vi "Camera.vi"(0 "Camera in":refnum<class "Camera.lvclass">, 1 "Stop":bool, 4 "BCG Image Processing":T3={"Brightness"=128.0, "Contrast"=45.0, "Gamma"=1.0} {"Brightness" scale=0.0..400.0; "Contrast" scale=0.0..90.0; "Gamma" scale=0.005..5.0}, 5 "error in (no error)":errorcluster, 6 "Machine Vision":T5, 7 "Camera settings":T2={"Gamma"=1.0, "Gain"=7, "Sharpness"=0, "Contrast"=0.009999999999999995, "Exposure"=0.0004073180282999787} {"Exposure" min=0.000244140625 max=0.5 scale=0.0002..0.5; "Contrast" min=0.0 max=1.0 scale=0.001..1.0; "Sharpness" min=0 max=2 step=1 scale=0.0..2.0; "Gain" min=0 max=100 step=1 scale=0.1..100.0; "Gamma" min=0.01 max=10.0 scale=0.01..10.0}, 10 "Material":T4, 12 "Loop 0":bool, 13 "Override presets":bool) -> (11 "Radius (Real-World)":dbl, 14 "Camera out":refnum<class "Camera.lvclass">, 15 "Average Strength":dbl, 16 "Global Report":T1 {"Mean Value" format="%.2f"; "%" format="%.2f"; "Area (calibrated)" format="%.2f"; "Maximal Value" format="%.2f"; "Minimal Value" format="%.2f"; "Standard Variation" format="%.2f"}, 17 "Image":T6(plugin-control), 18 "Camera":dbl[](array[numeric]), 19 "error out":errorcluster)   [LabVIEW 2021, in "Camera.lvclass"]
uses:
  Camera.lvclass
  Machine Vision.ctl
  Material.ctl
  Image processing.ctl
  Camera settings.ctl
  <vilib>/Utility/file.llb/Read Delimited Spreadsheet (string).vi
  <vilib>/vision/NI_Vision_Development_Module.lvlib
panel:
  out "Y":sgl
  out "X":sgl
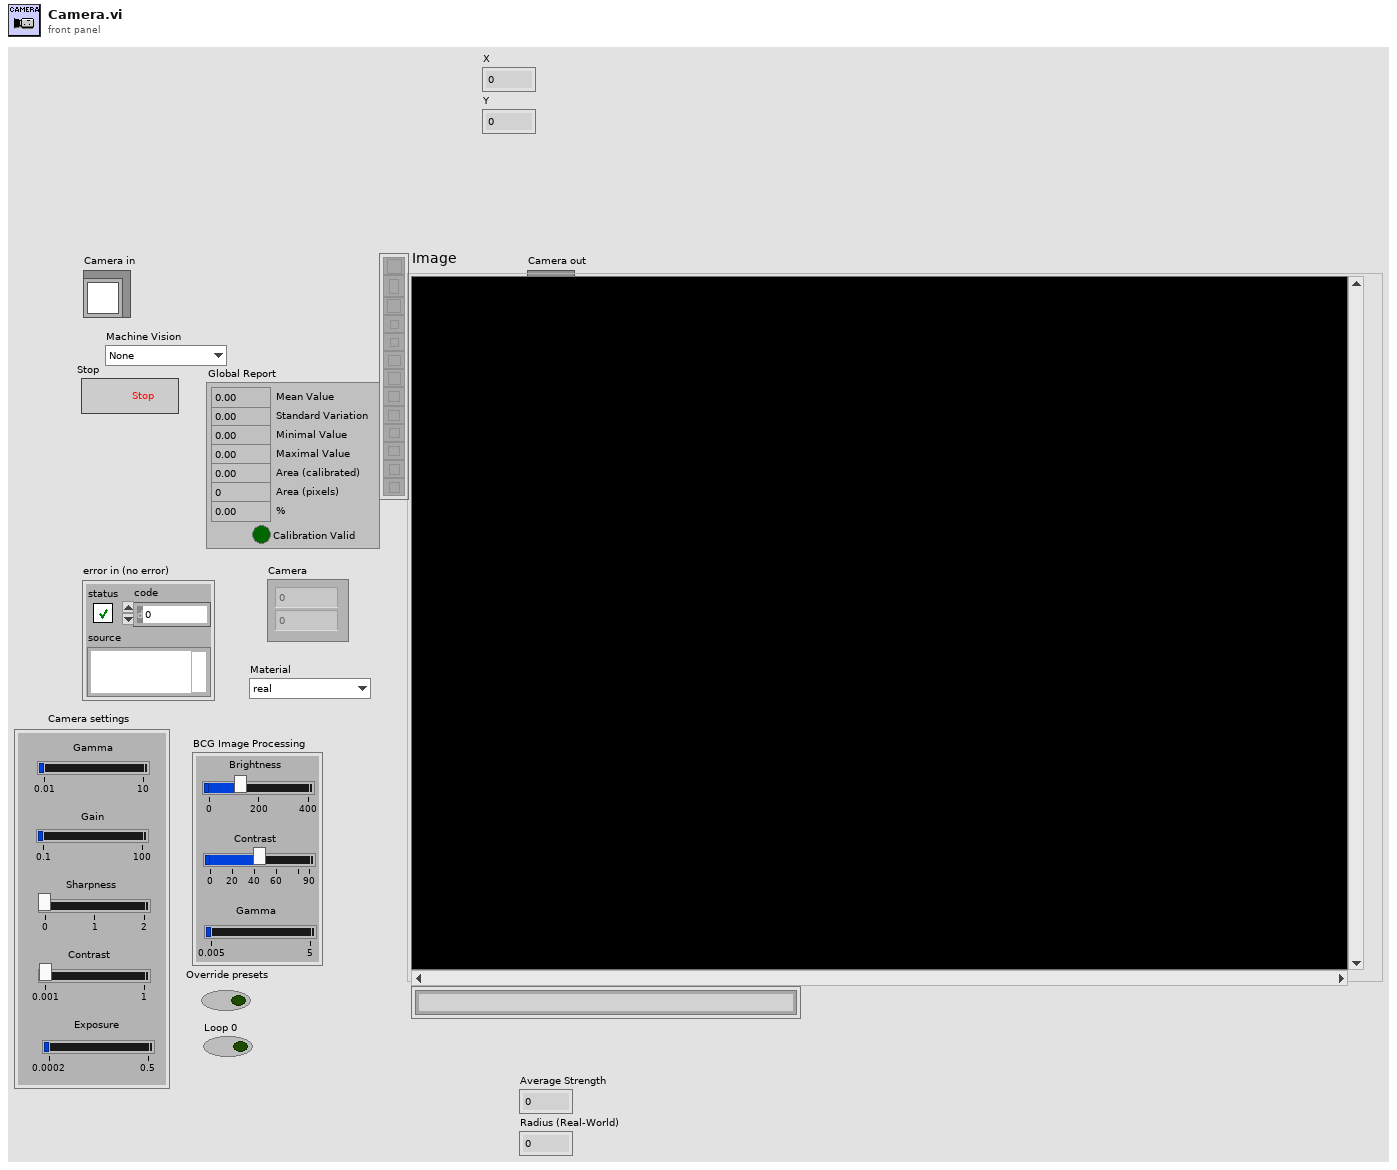
[diagram p1: front panel]
types:
  T1 = cluster{"Mean Value":sgl, "Standard Variation":sgl, "Minimal Value":sgl, "Maximal Value":sgl, "Area (calibrated)":sgl, "Area (pixels)":u32, "%":sgl, "Calibration Valid":bool}
  T2 = typedef "Camera.lvclass/Camera settings.ctl" = cluster{"Gamma":dbl, "Gain":i64, "Sharpness":i64, "Contrast":dbl, "Exposure":dbl}
  T3 = typedef "Camera.lvclass/Image processing.ctl" = cluster{"Brightness":sgl, "Contrast":sgl, "Gamma":sgl}
  T4 = typedef "Camera.lvclass/Material.ctl" = enum16{"real", "dummy", "PETG"}
  T5 = typedef "Camera.lvclass/Machine Vision.ctl" = enum16{"None", "Tray Fiducials", "Sensor Fiducials", "HPK Silicon", "Partial Hexaboard", "Partial Hexaboard Test", "100um dot", "Hexaboard", "Corner (TL, BR)", "Corner (BL, TR)", "V3 Sensor Cross", "V3 Sensor Circle", "test"}
  T6 = typedef "IMAQ Image.ctl" = refnum<image>
  T7 = typedef "File Paths.ctl" = cluster{"Glue Pattern Folder":path, "Carrier Tray Folder":path, "Pick Up Tool Fixture Folder":path, "Components Folder":path, "Bellows Tool Offset.txt":path, "Pick Up Tool Offset.txt":path, "Dispense Tip Offset.txt":path, "Log Files":path, "Gantry Assembly Map.txt":path, "Syringe and offset map.txt":path, "Controllers Folder":path, "Local dbase config":path}
  T8 = cluster{"Center (Pixels)":cluster{"X":sgl, "Y":sgl}, "Radius (Pixels)":dbl, "Center (Real-World)":cluster{"X":sgl, "Y":sgl}, "Radius (Real-World)":dbl, "Roundness (Real-World)":dbl, "Average Strength":dbl, "Average SNR (dB)":dbl}
  T9 = typedef "Edge New.ctl" = cluster{"Location (Pixel)":cluster{"X":sgl, "Y":sgl}, "Location (Real-World)":cluster{"X":sgl, "Y":sgl}, "Distance (Pixel)":dbl, "Distance (Real-World)":dbl, "Strength":dbl, "Noise":dbl, "Rising?":bool}
  T10 = cluster{"output string":sgl, "output string":sgl}
  T11 = typedef "ROI Descriptor" = cluster{"Global Rectangle":i32[], "Contours":cluster{"ID":enum32{"External", "Internal"}, "Type":u32, "Coordinates":i32[]}[]}
  T12 = typedef "Image Type" = u32
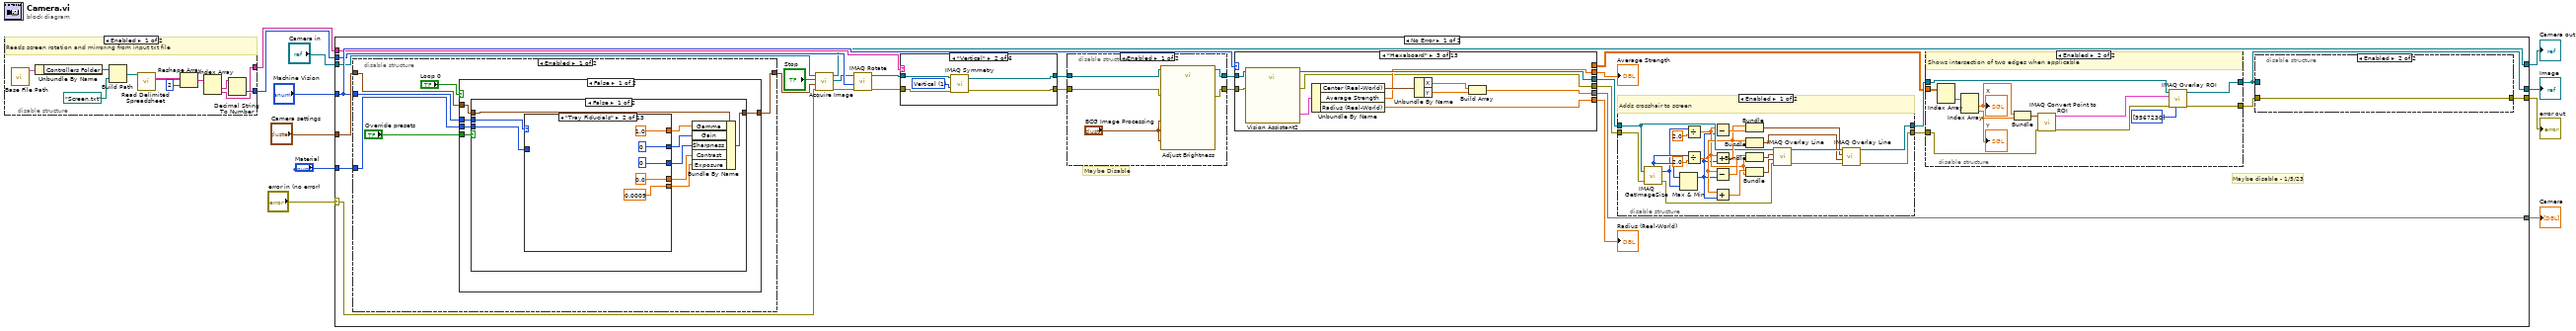
[diagram p0: block diagram]
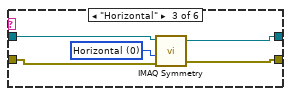
[diagram p4: hidden frame]
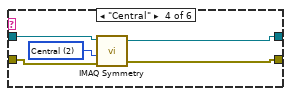
[diagram p5: hidden frame]
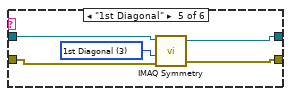
[diagram p6: hidden frame]
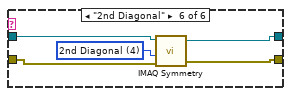
[diagram p7: hidden frame]
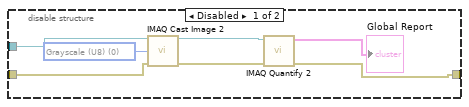
[diagram p8: hidden frame]
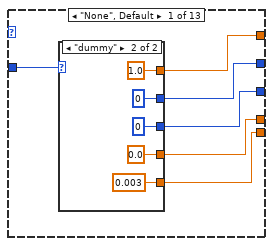
[diagram p12: hidden frame]
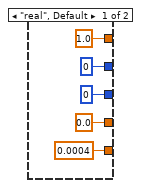
[diagram p13: hidden frame]
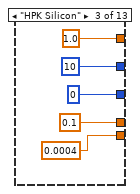
[diagram p14: hidden frame]
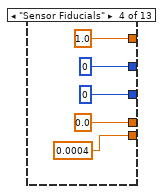
[diagram p15: hidden frame]
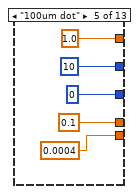
[diagram p16: hidden frame]
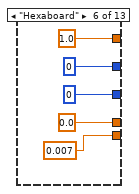
[diagram p17: hidden frame]
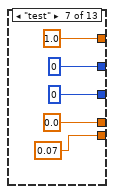
[diagram p18: hidden frame]
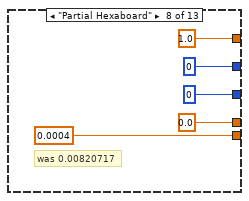
[diagram p19: hidden frame]
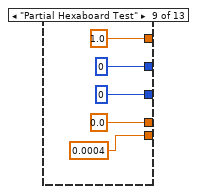
[diagram p20: hidden frame]
diagram:
  n1 = disable-structure shown="Enabled" {
    disable-tunnel: [w13 _] -> w2
    disable-tunnel: [w12 _] -> w1
    frame Enabled {
      # "Reads screen rotation and mirroring from input txt file"
      n2 = call "Base File Path.vi"() -> ("Paths Out"=w21:T7)  [unwired: 11 in]
      n3 = Unbundle By Name(w21) -> ("Controllers Folder"=w20:path)
      n4 = Build Path(base path=w20, name or relative path=path "Screen.txt") -> (appended path=w18:path)
      n5 = call-poly <vilib>:"Read Delimited Spreadsheet.vi"("file path (dialog if empty)"=w18) -> ("all rows"=w17:string[][])  [unwired: 9 in, 5 out]
      n6 = Reshape Array(w17, 2 ("dimension size")) -> (w15:string[])
      n7 = Index Array(array=w15) -> (element #1=w14:string, element #2=w12:string)  [unwired: 2 in]
      n8 = Decimal String To Number(string=w14) -> (number=w13:i32)  [unwired: 2 in, 1 out]
    }
    frame Disabled {
    }
  }
  n9 = case shown="No Error" "error in (no error)" {
    selector: "error in (no error)" -> [w24 w374]
    tunnel: [w31 w374] -> w10
    tunnel: [w27 w373] -> w9
    tunnel: "Camera in" -> [w28 w373]
    tunnel: [w50 _] -> w7
    tunnel: [w33 _] -> w6
    tunnel: "Machine Vision" -> [w48 _]
    tunnel: "Camera settings" -> [w49 _]
    tunnel: "Material" -> [w47 _]
    tunnel: w2 -> [w30 _]
    tunnel: w1 -> [w29 _]
    frame No Error {
      # "Maybe Disable"
      # "Maybe disable - 1/5/23"
      n10 = disable-structure shown="Enabled" {
        disable-tunnel: w48 -> [w136 _]
        disable-tunnel: w49 -> [w135 w235]
        disable-tunnel: [w134 w235] -> w25
        disable-tunnel: w47 -> [w131 _]
        frame Enabled {
          n11 = case shown="False" "Loop 0" {
            tunnel: "Override presets" -> [w141 _]
            tunnel: w136 -> [w140 _]
            tunnel: w135 -> [w139 w234]
            tunnel: [w138 w233] -> w134
            tunnel: w131 -> [w137 _]
            frame False {
              n12 = case shown="False" w141 {
                tunnel: w140 -> [w150 _]
                tunnel: w139 -> [w149 w227]
                tunnel: [w143 w227] -> w138
                tunnel: w137 -> [w142 _]
                frame False {
                  n13 = case shown="\"Tray Fiducials\"" w150 {
                    tunnel: [w155 1.0 ("Gamma::Value") 1.0 ("Gamma::Value") 1.0 ("Gamma::Value") 1.0 ("Gamma::Value") 1.0 ("Gamma::Value") 1.0 ("Gamma::Value") 1.0 ("Gamma::Value") 1.0 ("Gamma::Value") 1.0 ("Gamma::Value") 1.0 ("Gamma::Value") 1.0 ("Gamma::Value") 1.0 ("Gamma::Value")] -> w148
                    tunnel: [w151 i64 0 ("Gain::Value") i64 10 ("Gain::Value") i64 0 ("Gain::Value") i64 10 ("Gain::Value") i64 0 ("Gain::Value") i64 0 ("Gain::Value") i64 0 ("Gain::Value") i64 0 ("Gain::Value") i64 10 ("Gain::Value") i64 0 ("Gain::Value") i64 0 ("Gain::Value") i64 0 ("Gain::Value")] -> w147
                    tunnel: [w152 i64 0 ("Sharpness::Value") i64 0 ("Sharpness::Value") i64 0 ("Sharpness::Value") i64 0 ("Sharpness::Value") i64 0 ("Sharpness::Value") i64 0 ("Sharpness::Value") i64 0 ("Sharpness::Value") i64 0 ("Sharpness::Value") i64 0 ("Sharpness::Value") i64 0 ("Sharpness::Value") i64 0 ("Sharpness::Value") i64 0 ("Sharpness::Value")] -> w146
                    tunnel: [w153 0.0 ("Contrast::Value") 0.1 ("Contrast::Value") 0.0 ("Contrast::Value") 0.1 ("Contrast::Value") 0.0 ("Contrast::Value") 0.0 ("Contrast::Value") 0.0 ("Contrast::Value") 0.0 ("Contrast::Value") 0.075 ("Contrast::Value") 0.0 ("Contrast::Value") 0.0 ("Contrast::Value") 0.0 ("Contrast::Value")] -> w145
                    tunnel: [w154 0.0009 ("Exposure::Value") 0.0004 ("Exposure::Value") 0.0004 ("Exposure::Value") 0.0004 ("Exposure::Value") 0.007 ("Exposure::Value") 0.07 ("Exposure::Value") 0.0004 ("Exposure::Value") 0.0004 ("Exposure::Value") 0.0004 ("Exposure::Value") 0.007 ("Exposure::Value") 0.007 ("Exposure::Value") 0.001 ("Exposure::Value")] -> w144
                    tunnel: w142 -> [w156 _ _ _ _ _ _ _ _ _ _ _ _]
                    frame "None", Default {
                      n14 = case shown="\"dummy\"" w156 {
                        tunnel: [1.0 ("Gamma::Value") 1.0 ("Gamma::Value")] -> w155
                        tunnel: [0.0004 ("Exposure::Value") 0.003 ("Exposure::Value")] -> w154
                        tunnel: [0.0 ("Contrast::Value") 0.0 ("Contrast::Value")] -> w153
                        tunnel: [i64 0 ("Sharpness::Value") i64 0 ("Sharpness::Value")] -> w152
                        tunnel: [i64 0 ("Gain::Value") i64 0 ("Gain::Value")] -> w151
                        frame "real", Default {
                        }
                        frame "dummy" {
                        }
                      }
                    }
                    frame "Tray Fiducials" {
                    }
                    frame "HPK Silicon" {
                    }
                    frame "Sensor Fiducials" {
                    }
                    frame "100um dot" {
                    }
                    frame "Hexaboard" {
                    }
                    frame "test" {
                    }
                    frame "Partial Hexaboard" {
                      # "was 0.00820717"
                    }
                    frame "Partial Hexaboard Test" {
                    }
                    frame "Corner (TL, BR)" {
                    }
                    frame "Corner (BL, TR)" {
                    }
                    frame "V3 Sensor Cross" {
                    }
                    frame "V3 Sensor Circle" {
                    }
                  }
                  n15 = Bundle By Name(cluster=w149, "Gamma"=w148, "Gain"=w147, "Sharpness"=w146, "Contrast"=w145, "Exposure"=w144) -> (w143:T2)
                }
                frame True {
                }
              }
            }
            frame True {
              n16 = Bundle By Name(cluster=w234, "Gamma"=1.0, "Gain"=i64 0, "Sharpness"=i64 0, "Contrast"=0.0, "Exposure"=0.0004) -> (w233:T2)
            }
          }
        }
        frame Disabled {
        }
      }
      n17 = call-dynamic "Acquire Image.vi"("error in (no error)"=w24, "Cluster"=w25, "Stop"="Stop", "Camera in"=w28) -> ("error out"=w23:errorcluster, "Image Out"=w22:T6, "Camera out"=w27:refnum<class "Camera.lvclass">)  [unwired: 5 in]
      n18 = call "IMAQ Rotate"("error in (no error)"=w23, "Angle (degrees)"=w30, "Image Src"=w22) -> ("error out"=w35:errorcluster, "Image Dst Out"=w34:T6)  [unwired: 7 in]
      n19 = case shown="\"Vertical\"" w29 {
        tunnel: [w52 w57 w62 w67 w72 w77] -> w46
        tunnel: [w51 w56 w61 w66 w71 w76] -> w39
        tunnel: w35 -> [w51 w55 w60 w65 w70 w75]
        tunnel: w34 -> [w52 w54 w59 w64 w69 w74]
        frame "None", Default {
        }
        frame "Vertical" {
          w53 = u32 1 items=["Horizontal", "Vertical", "Central", "1st Diagonal", "2nd Diagonal"] ("Type of Symmetry")
          n20 = call "IMAQ Symmetry"("error in (no error)"=w55, "Type of Symmetry"=w53, "Image Src"=w54) -> ("error out"=w56:errorcluster, "Image Dst Out"=w57:T6)  [unwired: 2 in]
        }
        frame "Horizontal" {
          w58 = u32 0 items=["Horizontal", "Vertical", "Central", "1st Diagonal", "2nd Diagonal"] ("Type of Symmetry")
          n21 = call "IMAQ Symmetry"("error in (no error)"=w60, "Type of Symmetry"=w58, "Image Src"=w59) -> ("error out"=w61:errorcluster, "Image Dst Out"=w62:T6)  [unwired: 2 in]
        }
        frame "Central" {
          w63 = u32 2 items=["Horizontal", "Vertical", "Central", "1st Diagonal", "2nd Diagonal"] ("Type of Symmetry")
          n22 = call "IMAQ Symmetry"("error in (no error)"=w65, "Type of Symmetry"=w63, "Image Src"=w64) -> ("error out"=w66:errorcluster, "Image Dst Out"=w67:T6)  [unwired: 2 in]
        }
        frame "1st Diagonal" {
          w68 = u32 3 items=["Horizontal", "Vertical", "Central", "1st Diagonal", "2nd Diagonal"] ("Type of Symmetry")
          n23 = call "IMAQ Symmetry"("error in (no error)"=w70, "Type of Symmetry"=w68, "Image Src"=w69) -> ("error out"=w71:errorcluster, "Image Dst Out"=w72:T6)  [unwired: 2 in]
        }
        frame "2nd Diagonal" {
          w73 = u32 4 items=["Horizontal", "Vertical", "Central", "1st Diagonal", "2nd Diagonal"] ("Type of Symmetry")
          n24 = call "IMAQ Symmetry"("error in (no error)"=w75, "Type of Symmetry"=w73, "Image Src"=w74) -> ("error out"=w76:errorcluster, "Image Dst Out"=w77:T6)  [unwired: 2 in]
        }
      }
      n25 = disable-structure shown="Enabled" {
        disable-tunnel: w46 -> [w128 w129]
        disable-tunnel: [w126 w129] -> w45
        disable-tunnel: w39 -> [w125 w130]
        disable-tunnel: [w124 w130] -> w38
        frame Enabled {
          n26 = call "Adjust Brightness"("Image In"=w128, "Red BCG Values (Brightness 1)"="BCG Image Processing", "Green BCG Values (Brightness 1)"="BCG Image Processing", "Blue BCG Values (Brightness 1)"="BCG Image Processing", "error in"=w125) -> ("Image Out"=w126:T6, "error out"=w124:errorcluster)  [unwired: 21 in]
        }
        frame Disabled {
        }
      }
      n27 = case shown="\"Hexaboard\"" w48 {
        tunnel: [w240 w250 w258 w269 w280 w291 w302 w313 w322 w333 w344 w350 w362] -> w50
        tunnel: [w242 w252 w259 w270 w281 w292 w303 w315 w323 w334 w345 w354 w366] -> w44
        tunnel: w45 -> [w243 w252 w257 w268 w279 w290 w301 w312 w320 w331 w342 w355 w367]
        tunnel: [w238 0.0 ("Radius (Real-World)") w255 w266 w277 w288 w299 0.0 ("Radius (Real-World)") w319 w330 w341 0.0 ("Radius (Real-World)") 0.0 ("Radius (Real-World)")] -> w42
        tunnel: [w239 0.0 ("Strength") w256 w267 w278 w289 w300 _ w318 w329 w340 w360 w372] -> w41
        tunnel: [_ _ _ _ _ _ _ w311 _ _ _ _ _] -> w40
        tunnel: w38 -> [w237 w251 w253 w264 w275 w286 w297 w310 w317 w328 w339 w353 w365]
        tunnel: [w236 w251 w254 w265 w276 w287 w298 w309 w316 w327 w338 w352 w364] -> w37
        frame "Tray Fiducials", Default {
          n28 = call "Vision Assistant"("Image In"=w243, "error in"=w237) -> ("Image Out"=w242:T6, "Fitted Circle (Find Circular Edge 1)"=w241:T8, "error out"=w236:errorcluster)  [unwired: 23 in]
          n29 = Unbundle By Name(w241) -> ("Center (Real-World)"=w244:cluster{"X":sgl, "Y":sgl}, "Average Strength"=w239:dbl, "Radius (Real-World)"=w238:dbl)
          n30 = Unbundle By Name(w244) -> ("X"=w246:sgl, "Y"=w245:sgl)
          n31 = Build Array(w246, w245) -> (w240:sgl[])
        }
        frame "None" {
          n32 = Initialize Array(0.0 ("element")) -> (w250:dbl[])  [unwired: 1 in]
        }
        frame "Hexaboard" {
          n33 = call "Vision Assistant2"("Image In"=w257, "error in"=w253) -> ("Image Out"=w259:T6, "Fitted Circle (Find Circular Edge 1)"=w261:T8, "error out"=w254:errorcluster)  [unwired: 23 in]
          n34 = Unbundle By Name(w261) -> ("Center (Real-World)"=w263:cluster{"X":sgl, "Y":sgl}, "Average Strength"=w256:dbl, "Radius (Real-World)"=w255:dbl)
          n35 = Unbundle By Name(w263) -> ("X"=w262:sgl, "Y"=w260:sgl)
          n36 = Build Array(w262, w260) -> (w258:sgl[])
        }
        frame "test" {
          n37 = call "Vision Assistant11"("Image In"=w268, "error in"=w264) -> ("Image Out"=w270:T6, "Fitted Circle (Find Circular Edge 1)"=w272:T8, "error out"=w265:errorcluster)  [unwired: 23 in]
          n38 = Unbundle By Name(w272) -> ("Center (Real-World)"=w274:cluster{"X":sgl, "Y":sgl}, "Average Strength"=w267:dbl, "Radius (Real-World)"=w266:dbl)
          n39 = Unbundle By Name(w274) -> ("X"=w273:sgl, "Y"=w271:sgl)
          n40 = Build Array(w273, w271) -> (w269:sgl[])
        }
        frame "V3 Sensor Circle" {
          n41 = call "Vision Assistant4"("Image In"=w279, "error in"=w275) -> ("Image Out"=w281:T6, "Fitted Circle (Find Circular Edge 1)"=w283:T8, "error out"=w276:errorcluster)  [unwired: 23 in]
          n42 = Unbundle By Name(w283) -> ("Center (Real-World)"=w285:cluster{"X":sgl, "Y":sgl}, "Average Strength"=w278:dbl, "Radius (Real-World)"=w277:dbl)
          n43 = Unbundle By Name(w285) -> ("X"=w284:sgl, "Y"=w282:sgl)
          n44 = Build Array(w284, w282) -> (w280:sgl[])
        }
        frame "Partial Hexaboard" {
          n45 = call "Vision Assistant20"("Image In"=w290, "error in"=w286) -> ("Image Out"=w292:T6, "Fitted Circle (Find Circular Edge 1)"=w294:T8, "error out"=w287:errorcluster)  [unwired: 23 in]
          n46 = Unbundle By Name(w294) -> ("Center (Real-World)"=w296:cluster{"X":sgl, "Y":sgl}, "Average Strength"=w289:dbl, "Radius (Real-World)"=w288:dbl)
          n47 = Unbundle By Name(w296) -> ("X"=w295:sgl, "Y"=w293:sgl)
          n48 = Build Array(w295, w293) -> (w291:sgl[])
        }
        frame "Partial Hexaboard Test" {
          n49 = call "Vision Assistant10"("Image In"=w301, "error in"=w297) -> ("Image Out"=w303:T6, "Fitted Circle (Find Circular Edge 1)"=w305:T8, "error out"=w298:errorcluster)  [unwired: 23 in]
          n50 = Unbundle By Name(w305) -> ("Center (Real-World)"=w307:cluster{"X":sgl, "Y":sgl}, "Average Strength"=w300:dbl, "Radius (Real-World)"=w299:dbl)
          n51 = Unbundle By Name(w307) -> ("X"=w306:sgl, "Y"=w304:sgl)
          n52 = Build Array(w306, w304) -> (w302:sgl[])
        }
        frame "Corner (TL, BR)" {
          n53 = call "Vision Assistant3"("Image In"=w312, "error in"=w310) -> ("Image Out"=w315:T6, "error out"=w309:errorcluster, "Caliper Results (Top Left, Bottom Right)"=w311:sgl[][], "Calibrated Results (Top Left, Bottom Right)"=w314:sgl[][])  [unwired: 22 in]
          n54 = Index Array(array=w314) -> (element=w313:sgl[])  [unwired: 2 in]
        }
        frame "HPK Silicon" {
          n55 = call "Vision Assistant5"("Image In"=w320, "error in"=w317) -> ("Image Out"=w323:T6, "Fitted Circle (Find Circular Edge 1)"=w321:T8, "error out"=w316:errorcluster)  [unwired: 23 in]
          n56 = Unbundle By Name(w321) -> ("Center (Real-World)"=w326:cluster{"X":sgl, "Y":sgl}, "Average Strength"=w318:dbl, "Radius (Real-World)"=w319:dbl)
          n57 = Unbundle By Name(w326) -> ("X"=w325:sgl, "Y"=w324:sgl)
          n58 = Build Array(w325, w324) -> (w322:sgl[])
        }
        frame "Sensor Fiducials" {
          n59 = call "Vision Assistant9"("Image In"=w331, "error in"=w328) -> ("Image Out"=w334:T6, "Fitted Circle (Find Circular Edge 1)"=w332:T8, "error out"=w327:errorcluster)  [unwired: 23 in]
          n60 = Unbundle By Name(w332) -> ("Center (Real-World)"=w337:cluster{"X":sgl, "Y":sgl}, "Average Strength"=w329:dbl, "Radius (Real-World)"=w330:dbl)
          n61 = Unbundle By Name(w337) -> ("X"=w336:sgl, "Y"=w335:sgl)
          n62 = Build Array(w336, w335) -> (w333:sgl[])
        }
        frame "100um dot" {
          n63 = call "Vision Assistant6"("Image In"=w342, "error in"=w339) -> ("Image Out"=w345:T6, "Fitted Circle (Find Circular Edge 1)"=w343:T8, "error out"=w338:errorcluster)  [unwired: 23 in]
          n64 = Unbundle By Name(w343) -> ("Center (Real-World)"=w348:cluster{"X":sgl, "Y":sgl}, "Average Strength"=w340:dbl, "Radius (Real-World)"=w341:dbl)
          n65 = Unbundle By Name(w348) -> ("X"=w347:sgl, "Y"=w346:sgl)
          n66 = Build Array(w347, w346) -> (w344:sgl[])
        }
        frame "Corner (BL, TR)" {
          n67 = call "Vision Assistant7"("Image In"=w355, "error in"=w353) -> ("Image Out"=w354:T6, "Used Edges (Adv. Straight Edge 1)"=w359:cluster{"Edge Information":T9[]}[], "error out"=w352:errorcluster)  [unwired: 23 in]
          n68 = Index Array(array=w359) -> (element=w358:cluster{"Edge Information":T9[]})  [unwired: 1 in]
          n69 = Unbundle By Name(w358) -> ("Edge Information"=w357:T9[])
          n70 = Index Array(array=w357) -> (element=w356:T9)  [unwired: 1 in]
          n71 = Unbundle(w356) -> ("Location (Real-World)"=w351:cluster{"X":sgl, "Y":sgl}, "Strength"=w360:dbl)  [unwired: 5 out]
          n72 = Cluster To Array(cluster=w351) -> (array=w350:sgl[])
        }
        frame "V3 Sensor Cross" {
          n73 = call "Vision Assistant8"("Image In"=w367, "error in"=w365) -> ("Image Out"=w366:T6, "Used Edges (Adv. Straight Edge 1)"=w371:cluster{"Edge Information":T9[]}[], "error out"=w364:errorcluster)  [unwired: 23 in]
          n74 = Index Array(array=w371) -> (element=w370:cluster{"Edge Information":T9[]})  [unwired: 1 in]
          n75 = Unbundle By Name(w370) -> ("Edge Information"=w369:T9[])
          n76 = Index Array(array=w369) -> (element=w368:T9)  [unwired: 1 in]
          n77 = Unbundle(w368) -> ("Location (Real-World)"=w363:cluster{"X":sgl, "Y":sgl}, "Strength"=w372:dbl)  [unwired: 5 out]
          n78 = Cluster To Array(cluster=w363) -> (array=w362:sgl[])
        }
      }
      "Radius (Real-World)" <- w42
      "Average Strength" <- w41
      n79 = disable-structure shown="Enabled" {
        disable-tunnel: w44 -> [w109 w123]
        disable-tunnel: [w112 w123] -> w43
        disable-tunnel: w37 -> [w108 w122]
        disable-tunnel: [w110 w122] -> w36
        frame Enabled {
          # "Adds crosshair to screen"
          n80 = call "IMAQ GetImageSize"("Image"=w109, "error in (no error)"=w108) -> ("Y Resolution"=w101:i32, "X Resolution"=w102:i32, "error out"=w107:errorcluster)  [unwired: 2 in]
          n81 = Max & Min(x=w102, y=w101) -> (max(x,y)=w100:i32)  [unwired: 1 out]
          n82 = Divide(x=w101, y=2.0) -> (x/y=w103:dbl)
          n83 = Divide(x=w102, y=2.0) -> (x/y=w104:dbl)
          n84 = Subtract(x=w103, y=w100) -> (x-y=w117:dbl)
          n85 = Add(x=w103, y=w100) -> (x+y=w118:dbl)
          n86 = Subtract(x=w104, y=w100) -> (x-y=w113:dbl)
          n87 = Add(x=w104, y=w100) -> (x+y=w114:dbl)
          n88 = Bundle(w104, w117) -> (w119:cluster{dbl, dbl})  [unwired: 1 in]
          n89 = Bundle(w104, w118) -> (w120:cluster{dbl, dbl})  [unwired: 1 in]
          n90 = Bundle(w113, w103) -> (w116:cluster{dbl, dbl})  [unwired: 1 in]
          n91 = Bundle(w114, w103) -> (w115:cluster{dbl, dbl})  [unwired: 1 in]
          n92 = call "IMAQ Overlay Line"("error in (no error)"=w107, "End Point"=w115, "Start Point"=w116, "Image"=w109) -> ("error out"=w111:errorcluster, "Image Out"=w121:T6)  [unwired: 6 in]
          n93 = call "IMAQ Overlay Line"("error in (no error)"=w111, "End Point"=w120, "Start Point"=w119, "Image"=w121) -> ("error out"=w110:errorcluster, "Image Out"=w112:T6)  [unwired: 6 in]
        }
        frame Disabled {
        }
      }
      n94 = disable-structure shown="Enabled" {
        disable-tunnel: [w87 w95] -> w33
        disable-tunnel: w43 -> [w87 w94]
        disable-tunnel: w40 -> [_ w93]
        disable-tunnel: w36 -> [w86 w90]
        disable-tunnel: [w86 w88] -> w32
        frame Disabled {
        }
        frame Enabled {
          # "Shows intersection of two edges when applicable"
          n95 = Index Array(array=w93) -> (element=w92:sgl[])  [unwired: 2 in]
          n96 = Index Array(array=w92) -> (element #1=w96:sgl, element #2=w98:sgl)  [unwired: 2 in]
          "X" <- w96
          "Y" <- w98
          n97 = Bundle("output string"=w96, "output string"=w98) -> (w99:T10)  [unwired: 1 in]
          n98 = call "IMAQ Convert Point to ROI"("error in (no error)"=w90, "Point"=w99) -> ("error out"=w89:errorcluster, "ROI Descriptor"=w97:T11)  [unwired: 7 in]
          n99 = call "IMAQ Overlay ROI"("Colors (Green)"=u32[] [9567230], "error in (no error)"=w89, "ROI Descriptor"=w97, "Image"=w94) -> ("error out"=w88:errorcluster, "Image Out"=w95:T6)  [unwired: 6 in]
        }
      }
      n100 = disable-structure shown="Enabled" {
        disable-tunnel: w33 -> [w80 _]
        disable-tunnel: w32 -> [w82 w85]
        disable-tunnel: [w83 w85] -> w31
        frame Disabled {
          w79 = T12 0 items=["Grayscale (U8)", "Grayscale (I16)", "Grayscale (SGL)", "Complex (CSG)", "RGB (U32)", "HSL (U32)", "RGB (U64)", "Grayscale (U16)"] ("Image Type")
          n101 = call "IMAQ Cast Image 2"("Image Src"=w80, "Image Type"=w79, "error in (no error)"=w82) -> ("Image Dst Out"=w78:T6, "error out"=w81:errorcluster)  [unwired: 11 in]
          n102 = call "IMAQ Quantify 2"("error in (no error)"=w81, "Image"=w78) -> ("error out"=w83:errorcluster, "Global Report"=→"Global Report":T1)  [unwired: 7 in, 1 out]
        }
        frame Enabled {
        }
      }
    }
    frame Error {
    }
  }
  "error out" <- w10
  "Camera out" <- w9
  "Camera" <- w7
  "Image" <- w6
